vi "ResizePane.vi"(6 "buffer (10)":i16=10, 8 "error in (no error)":errorcluster, 10 "NewBnds":T1, 11 "Sudoku in":refnum<class "Sudoku.lvclass">) -> (0 "error out":errorcluster, 2 "Cell Size":i32, 3 "Sudoku out":refnum<class "Sudoku.lvclass">)   [LabVIEW 2021, in "Sudoku.lvclass"]
uses:
  Sudoku.lvclass
  <vilib>/Utility/miscctls.llb/LVRectTypeDef.ctl
  <vilib>/Utility/miscctls.llb/LVBoundsTypeDef.ctl
  Sudoku.lvclass/Sudoku.ctl
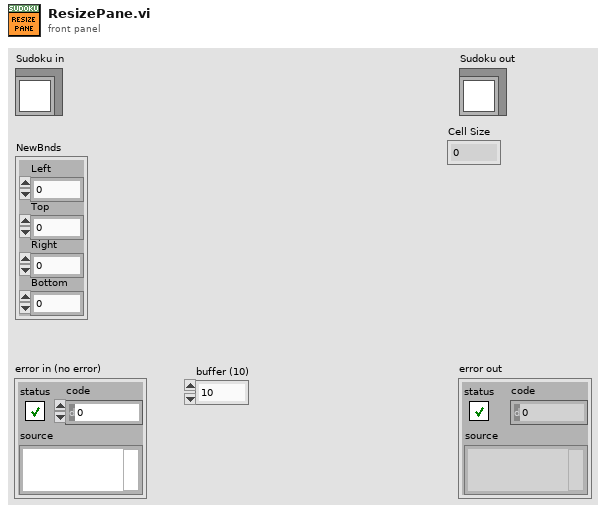
[diagram p1: front panel]
types:
  T1 = typedef "LVRectTypeDef.ctl" = cluster{"Left":i16, "Top":i16, "Right":i16, "Bottom":i16}
  T2 = typedef "LVBoundsTypeDef.ctl" = cluster{"Width":u32, "Height":u32}
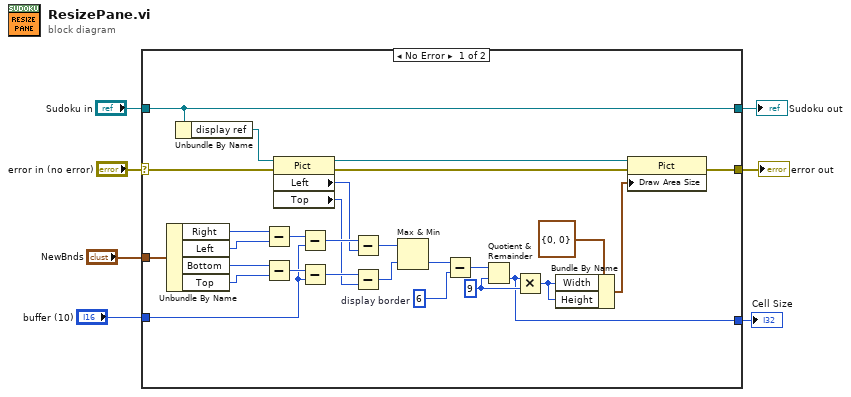
[diagram p0: block diagram]
diagram:
  n1 = case shown="No Error" "error in (no error)" {
    selector: "error in (no error)" -> [w33 w37]
    tunnel: [w9 w37] -> w6
    tunnel: [w34 w36] -> w4
    tunnel: "Sudoku in" -> [w34 w36]
    tunnel: "NewBnds" -> [w35 _]
    tunnel: "buffer (10)" -> [w25 _]
    tunnel: [w8 _] -> w1
    frame No Error {
      w15 = 9 ("y")
      w17 = 6  # display border
      n2 = Unbundle By Name(w35) -> ("Right"=w31:i16, "Left"=w30:i16, "Bottom"=w29:i16, "Top"=w28:i16)
      n3 = Unbundle By Name(w34) -> ("display ref"=w32:refnum<vi>)
      n4 = Subtract(x=w31, y=w30) -> (x-y=w26:i16)
      n5 = Subtract(x=w29, y=w28) -> (x-y=w27:i16)
      n6 = property class="Pict"(reference=w32, error in=w33) -> (reference out=w13:refnum<vi>, error out=w14:errorcluster, "Left"=w21:i32, "Top"=w22:i32)
      n7 = Subtract(x=w26, y=w25) -> (x-y=w24:i16)
      n8 = Subtract(x=w27, y=w25) -> (x-y=w23:i16)
      n9 = Subtract(x=w24, y=w21) -> (x-y=w20:i32)
      n10 = Subtract(x=w23, y=w22) -> (x-y=w19:i32)
      n11 = Max & Min(x=w20, y=w19) -> (min(x,y)=w18:i32)  [unwired: 1 out]
      n12 = Subtract(x=w18, y=w17) -> (x-y=w16:i32)
      n13 = Quotient & Remainder(x=w16, y=w15) -> (floor(x/y)=w8:i32)  [unwired: 1 out]
      n14 = Multiply(x=w8, y=w15) -> (x*y=w11:i32)
      n15 = Bundle By Name(cluster=T2 {"Width"=0, "Height"=0} ("Draw Area Size"), "Width"=w11, "Height"=w11) -> (w10:T2)
      n16 = property class="Pict"(reference=w13, error in=w14, "Draw Area Size"=w10) -> (error out=w9:errorcluster)  [unwired: 1 out]
    }
    frame Error {
    }
  }
  "error out" <- w6
  "Sudoku out" <- w4
  "Cell Size" <- w1
